vi "Begin.vi"(8 "error in":errorcluster) -> (0 "error out":errorcluster)   [LabVIEW 2016]
doc: "Called before other user functions, this VI is expected to open initial I/O refnums, load in file data, and do all program initialization. Notice that the <B>error out</B> terminal is simply used for data flow. Wiring it to other structures or subVIs ensures that this VI runs first."
uses:
  <vilib>/Rock Robotics/SystemInterfaces/DIO/FPGA_DIOPWMChannel.ctl
  <vilib>/Rock Robotics/WPI/SafetyOutput/WPI_SafetyOutputConfigMenu.ctl
  <vilib>/Rock Robotics/WPI/DriverStation/WPI_DriverStationRobotMode2.ctl
  <vilib>/Rock Robotics/WPI/Joystick/WPI_JoystickDeviceEnum.ctl
  <vilib>/Rock Robotics/SystemInterfaces/DIO/FPGA_DIOChannel.ctl
  <vilib>/Rock Robotics/WPI/Encoder/WPI_EncoderType.ctl
  NI WPI/WPI_SerialPort_USB.ctl
  <vilib>/Rock Robotics/WPI/ThirdParty/CanMotor/TalonSRX/WPI_CANTalonSRX_APIControlMode.ctl
  <vilib>/Rock Robotics/WPI/Solenoid/WPI_SolenoidChannel.ctl
  <vilib>/Rock Robotics/SystemInterfaces/i2clib/i2c_bus.ctl
  <vilib>/Rock Robotics/WPI/Solenoid/WPI_SolenoidValue.ctl
  Robot Global Data.vi
  <vilib>/Rock Robotics/Network Tables/NT Write String Array.vi
  <vilib>/Rock Robotics/WPI/Counter/WPI_CounterDigitalInputToDigitalSource.vi
  navX Library v2/IO/Open/Z900_navX_Open_Serial.vi
  <vilib>/Rock Robotics/WPI/Solenoid/WPI_SolenoidOpenSingle.vi
  <vilib>/Rock Robotics/WPI/MotorControl/WPI_MotorControlOpen VictorSP.vi
  <vilib>/Rock Robotics/WPI/RobotDrive/WPI_RobotDriveOpen4MotorWithVictorSP.vi
  <vilib>/Rock Robotics/WPI/Solenoid/WPI_SolenoidSetEnum.vi
  navX Library v2/navX Library v2.lvlib
  NI WPI/NI WPI Serial USB.lvlib
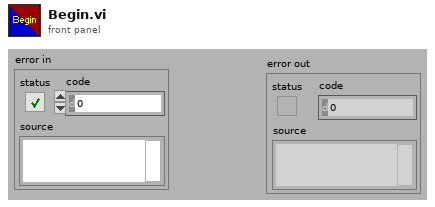
[diagram p1: front panel]
types:
  T1 = typedef "FPGA_DIOChannel.ctl" = enum8{"DIO 0", "DIO 1", "DIO 2", "DIO 3", "DIO 4", "DIO 5", "DIO 6", "DIO 7", "DIO 8", "DIO 9", "DIO MXP 0", "DIO MXP 1", "DIO MXP 2", "DIO MXP 3", "DIO MXP 4", "DIO MXP 5", "DIO MXP 6", "DIO MXP 7", "DIO MXP 8", "DIO MXP 9", "DIO MXP 10", "DIO MXP 11", "DIO MXP 12", "DIO MXP 13", "DIO MXP 14", "DIO MXP 15", "SPI Port CS1", "SPI Port CS2", "SPI Port CS3", "SPI Port MISO", "SPI Port MOSI", "Invalid"}
  T2 = typedef "WPI_SolenoidValue.ctl" = enum16{"Off", "On", "Forward", "Reverse"}
  T3 = typedef "i2c_bus.ctl" = enum16{"I2C On-Board", "I2C MXP", "Invalid"}
  T4 = typedef "WPI_SolenoidChannel.ctl" = enum8{"Solenoid 0", "Solenoid 1", "Solenoid 2", "Solenoid 3", "Solenoid 4", "Solenoid 5", "Solenoid 6", "Solenoid 7", "Invalid"}
  T5 = typedef "FPGA_DIOPWMChannel.ctl" = enum8{"PWM 0", "PWM 1", "PWM 2", "PWM 3", "PWM 4", "PWM 5", "PWM 6", "PWM 7", "PWM 8", "PWM 9", "PWM MXP 0", "PWM MXP 1", "PWM MXP 2", "PWM MXP 3", "PWM MXP 4", "PWM MXP 5", "PWM MXP 6", "PWM MXP 7", "PWM MXP 8", "PWM MXP 9", "Invalid"}
  T6 = typedef "WPI_JoystickDeviceEnum.ctl" = enum16{"USB 0", "USB 1", "USB 2", "USB 3", "USB 4", "USB 5"}
  T7 = typedef "WPI_CANTalonSRX_APIControlMode.ctl" = enum8{"Percent VBus", "Speed", "Position", "Slave", "Unchanged / Invalid", "Voltage Compensation", "Current", "Motion Profile", "Motion Magic"}
  T8 = typedef "NI WPI Serial USB.lvlib/WPI_SerialPort_USB.ctl" = enum16{"Onboard RS-232", "MXP TTL", "USB"}
  T9 = typedef "WPI_EncoderType.ctl" = enum16{"1x", "2x", "4x"}
  T10 = typedef "WPI_DriverStationRobotMode2.ctl" = enum16{"Autonomous Disabled", "Autonomous Enabled", "Teleop Disabled", "Teleop Enabled", "Disconnected", "Finish", "Test Disabled", "Test Enabled", "Emergency Stopped"}
  T11 = typedef "WPI_SafetyOutputConfigMenu.ctl" = enum16{"Enable", "Disable"}
  T12 = typedef "WPI_JoystickDevRef.ctl" = cluster{"Device":T6}
  T13 = typedef "WPI_I2CDevRef.ctl" = cluster{"DevStatus":errorcluster, "Device Address":u8, "Handle":i32, "I2C Bus":T3}
  T14 = typedef "WPI_MotorControlDeviceRef.ctl" = cluster{"DeviceStatus":errorcluster, "Type":T15, "PWM":cluster{"PWM Channel":T5, "DeadBand":T16}, "CAN":cluster{"Device Number":u8, "SetOutput VI Ref":variant, "GetOutput VI Ref":variant, "Enable VI Ref":variant, "Disable VI Ref":variant, "Data":variant}, "Invert":bool}
  T15 = typedef "WPI_MotorControlType.ctl" = enum16{"PWM", "CAN"}
  T16 = typedef "WPI_PWMDeadband.ctl" = cluster{"Name":string, "maxPositivePwm":i32, "minPositivePwm":i32, "centerPwm":i32, "maxNegativePwm":i32, "minNegativePwm":i32, "angularRange":u16}
  T17 = typedef "WPI_RobotDriveDevRef.ctl" = cluster{"DevStatus":errorcluster, "Motors[]":T14[], "Square Inputs":bool, "Max Output":dbl}
  T18 = typedef "WPI_DigitalInputDevRef.ctl" = cluster{"DevStatus":errorcluster, "DIO Channel":T1}
  T19 = typedef "FPGA_CounterEncoderSourceConvertionLVSourceType.ctl" = cluster{"DevStatus":errorcluster, "AnalogTriggerMode?":bool, "DigitalMode":cluster{"DIO Channel":T20}, "AnalogTriggerMode":cluster{"AnalogTriggerIndex":T21, "OutputType":T22}}
  T20 = typedef "FPGA_DIODigitalSourceChannel.ctl" = enum8{"DIO 0", "DIO 1", "DIO 2", "DIO 3", "DIO 4", "DIO 5", "DIO 6", "DIO 7", "DIO 8", "DIO 9", "DIO MXP 0", "DIO MXP 1", "DIO MXP 2", "DIO MXP 3", "DIO MXP 4", "DIO MXP 5", "DIO MXP 6", "DIO MXP 7", "DIO MXP 8", "DIO MXP 9", "DIO MXP 10", "DIO MXP 11", "DIO MXP 12", "DIO MXP 13", "DIO MXP 14", "DIO MXP 15", "Disabled"}
  T21 = typedef "FPGA_AnalogTriggerIndex.ctl" = enum8{"Trig 0", "Trig 1", "Trig 2", "Trig 3", "Trig 4", "Trig 5", "Trig 6", "Trig 7", "Invalid"}
  T22 = typedef "FPGA_AnalogTriggerOutType.ctl" = enum16{"InWindow", "TriggerState", "Rising", "Falling"}
  T23 = typedef "WPI_EncoderDevRef.ctl" = cluster{"DevStatus":errorcluster, "EncoderIndex":T24, "CounterIndex":T25, "DistancePerCount":dbl, "Decoding Type":T9}
  T24 = typedef "FPGA_EncoderIdx.ctl" = enum8{"Enc 0", "Enc 1", "Enc 2", "Enc 3", "Enc 4", "Enc 5", "Enc 6", "Enc 7", "Invalid"}
  T25 = typedef "FPGA_CounterCtrSystemIndex.ctl" = enum8{"Ctr 0", "Ctr 1", "Ctr 2", "Ctr 3", "Ctr 4", "Ctr 5", "Ctr 6", "Ctr 7", "Invalid"}
  T26 = typedef "navX Library v2.lvlib/Z900_navX_DeviceTypeDef.ctl" = cluster{"Interface":cluster{"Protocol":T27, "Update Rate (4Hz-100Hz)":u8, "navX Open TypeDef":variant}, "Notify Packet":refnum<notifier>, "Loop VI Refnum":refnum<vi>, "Ready to Close Occurrence Refnum":refnum<k4>}
  T27 = typedef "navX Library v2.lvlib/Z900_navX_ProtocolTypeDef.ctl" = enum16{"SERIAL", "I2C", "SPI"}
  T28 = typedef "WPI_SolenoidDevRef.ctl" = cluster{"DevStatus":errorcluster, "Pneumatics Control Module":u8, "Forward Solenoid Channel":T4, "Reverse Solenoid Channel":T4}
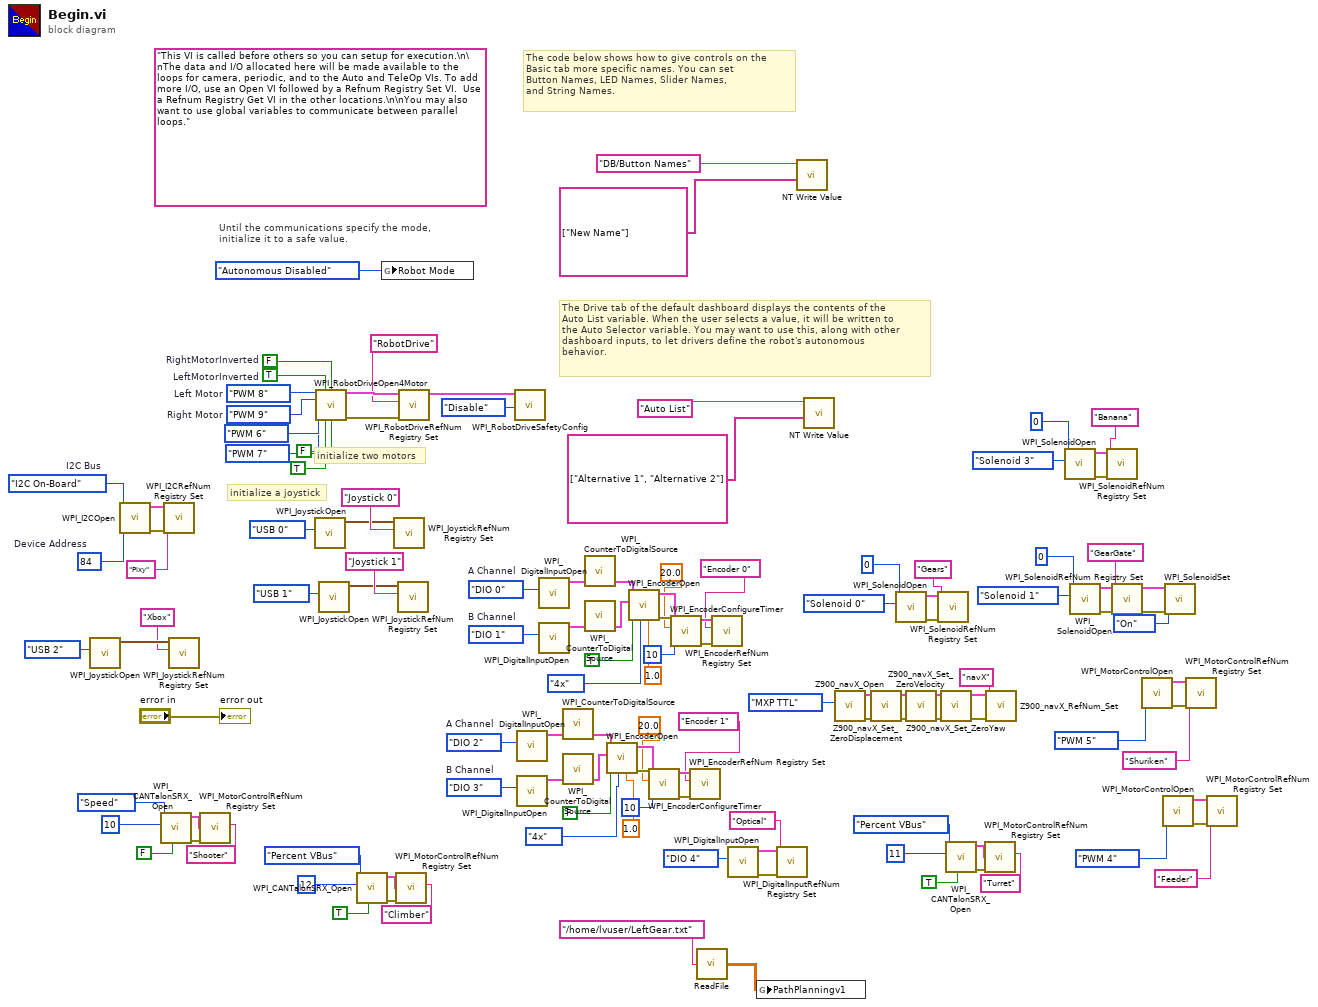
[diagram p0: block diagram]
diagram:
  w14 = u8 84  # Device Address
  w15 = i2c_bus."I2C On-Board"  # I2C Bus
  w88 = FPGA_DIOChannel."DIO 3"  # B Channel
  w87 = FPGA_DIOChannel."DIO 2"  # A Channel
  w104 = FPGA_DIOChannel."DIO 1"  # B Channel
  w103 = FPGA_DIOChannel."DIO 0"  # A Channel
  (unwired) "This VI is called before others so you can setup for execution.\n\nThe data and I/O allocated here will be made available to the loops for camera, periodic, and to the Auto and TeleOp VIs. To add more I/O, use an Open VI followed by a Refnum Registry Set VI.  Use a Refnum Registry Get VI in the other locations.\n\nYou may also want to use global variables to communicate between parallel loops."
  w119 = FPGA_DIOPWMChannel."PWM 9"  # Right Motor
  w120 = FPGA_DIOPWMChannel."PWM 8"  # Left Motor
  w124 = TRUE  # LeftMotorInverted
  w125 = FALSE  # RightMotorInverted
  # "The Drive tab of the default dashboard displays the contents of the\nAuto List variable. When the user selects a value, it will be written to\nthe Auto Selector variable. You may want to use this, along with other\ndashboard inputs, to let drivers define the robot's autonomous\nbehavior."
  # "The code below shows how to give controls on the\nBasic tab more specific names. You can set\nButton Names, LED Names, Slider Names,\nand String Names."
  # "initialize a joystick"
  # "Until the communications specify the mode,\ninitialize it to a safe value."
  # "initialize two motors"
  n1 = call <vilib>:"WPI_JoystickOpen.vi"("JoystickDevice"=WPI_JoystickDeviceEnum."USB 2") -> ("JoystickDevRef"=w28:T12)  [unwired: 10 in]
  n2 = call <vilib>:"WPI_I2COpen.vi"("Device Address"=w14, "I2C Bus"=w15) -> ("error out"=w13:errorcluster, "I2CDevRef"=w12:T13)  [unwired: 8 in]
  n3 = call <vilib>:"WPI_CANTalonSRX_Open.vi"("Invert"=FALSE, "Device Number"=10, "Control Mode"=WPI_CANTalonSRX_APIControlMode."Speed") -> ("error out"=w55:errorcluster, "CAN Talon SRX Ref"=w56:T14)  [unwired: 7 in]
  n4 = call <vilib>:"WPI_I2CRefNum Registry Set.vi"("error in (no error)"=w13, "refnum name"="Pixy", "I2CDevRef"=w12) -> ()  [unwired: 7 in, 2 out]
  n5 = call <vilib>:"WPI_JoystickRefNum Registry Set.vi"("refnum name"="Xbox", "JoystickDevRef"=w28) -> ()  [unwired: 8 in, 2 out]
  n6 = call <vilib>:"WPI_MotorControlRefNum Registry Set.vi"("error in (no error)"=w55, "refnum name"="Shooter", "MotorControlDevRef"=w56) -> ()  [unwired: 7 in, 2 out]
  n7 = call <vilib>:"WPI_JoystickOpen.vi"("JoystickDevice"=WPI_JoystickDeviceEnum."USB 0") -> ("JoystickDevRef"=w114:T12)  [unwired: 10 in]
  n8 = call-poly <vilib>:"WPI_RobotDriveOpen4Motor.vi"("Rear Left Motor"=w120, "Rear Left Motor Inverted"=w124, "Rear Right Motor Inverted"=w125, "Rear Right Motor"=w119, "Front Left Motor"=FPGA_DIOPWMChannel."PWM 6", "Front Right Motor"=FPGA_DIOPWMChannel."PWM 7", "Front Left Motor Inverted"=TRUE, "Front Right Motor Inverted"=FALSE) -> ("RobotDriveDevRef"=w123:T17, "error out"=w121:errorcluster)  [unwired: 6 in]
  n9 = call <vilib>:"WPI_JoystickOpen.vi"("JoystickDevice"=WPI_JoystickDeviceEnum."USB 1") -> ("JoystickDevRef"=w106:T12)  [unwired: 10 in]
  n10 = call <vilib>:"WPI_CANTalonSRX_Open.vi"("Invert"=TRUE, "Device Number"=12, "Control Mode"=WPI_CANTalonSRX_APIControlMode."Percent VBus") -> ("error out"=w49:errorcluster, "CAN Talon SRX Ref"=w50:T14)  [unwired: 7 in]
  n11 = global write "Robot Global Data.vi" "Robot Mode"(WPI_DriverStationRobotMode2."Autonomous Disabled" ("Robot Mode")) -> ()
  n12 = call <vilib>:"WPI_JoystickRefNum Registry Set.vi"("refnum name"="Joystick 0", "JoystickDevRef"=w114) -> ()  [unwired: 8 in, 2 out]
  n13 = call <vilib>:"WPI_MotorControlRefNum Registry Set.vi"("error in (no error)"=w49, "refnum name"="Climber", "MotorControlDevRef"=w50) -> ()  [unwired: 7 in, 2 out]
  n14 = call <vilib>:"WPI_JoystickRefNum Registry Set.vi"("refnum name"="Joystick 1", "JoystickDevRef"=w106) -> ()  [unwired: 8 in, 2 out]
  n15 = call <vilib>:"WPI_RobotDriveRefNum Registry Set.vi"("error in (no error)"=w121, "refnum name"="RobotDrive", "RobotDriveDevRef"=w123) -> ("RobotDriveDevRef"=w118:T17)  [unwired: 1 in, 7 out]
  n16 = call <vilib>:"WPI_RobotDriveSafetyConfig.vi"("mode"=WPI_SafetyOutputConfigMenu."Disable", "RobotDriveDevRef"=w118) -> ()  [unwired: 8 in, 2 out]
  n17 = call <vilib>:"WPI_DigitalInputOpen.vi"("DIO Channel"=w87) -> ("DigitalInputDevRef"=w84:T18)  [unwired: 1 in, 9 out]
  n18 = call <vilib>:"WPI_DigitalInputOpen.vi"("DIO Channel"=w88) -> ("DigitalInputDevRef"=w85:T18)  [unwired: 1 in, 9 out]
  n19 = call <vilib>:"WPI_DigitalInputOpen.vi"("DIO Channel"=w103) -> ("DigitalInputDevRef"=w100:T18)  [unwired: 1 in, 9 out]
  n20 = call <vilib>:"WPI_DigitalInputOpen.vi"("DIO Channel"=w104) -> ("DigitalInputDevRef"=w101:T18)  [unwired: 1 in, 9 out]
  n21 = call-poly <vilib>:"WPI_CounterToDigitalSource.vi"("DigitalInputDevRef"=w84) -> ("Digital Source"=w83:T19)  [unwired: 6 out]
  n22 = call-poly <vilib>:"WPI_CounterToDigitalSource.vi"("DigitalInputDevRef"=w85) -> ("Digital Source"=w86:T19)  [unwired: 6 out]
  n23 = call-poly <vilib>:"WPI_CounterToDigitalSource.vi"("DigitalInputDevRef"=w100) -> ("Digital Source"=w99:T19)  [unwired: 6 out]
  n24 = call-poly <vilib>:"WPI_CounterToDigitalSource.vi"("DigitalInputDevRef"=w101) -> ("Digital Source"=w102:T19)  [unwired: 6 out]
  n25 = call <vilib>:"WPI_EncoderOpen.vi"("DistancePerCount"=1.0, "Decoding Type"=WPI_EncoderType."4x", "Invert Direction (False)"=FALSE, "BSource"=w86, "ASource"=w83) -> ("error out"=w81:errorcluster, "EncoderDevRef"=w80:T23)  [unwired: 3 in, 2 out]
  n26 = call <vilib>:"WPI_EncoderOpen.vi"("DistancePerCount"=1.0, "Decoding Type"=WPI_EncoderType."4x", "Invert Direction (False)"=TRUE, "BSource"=w102, "ASource"=w99) -> ("error out"=w95:errorcluster, "EncoderDevRef"=w94:T23)  [unwired: 3 in, 2 out]
  n27 = call <vilib>:"WPI_EncoderConfigureTimer.vi"("error in (no error)"=w81, "Number Samples to Average"=u8 10, "Minimum Rate"=20.0, "EncoderDevRef"=w80) -> ("error out"=w77:errorcluster, "EncoderDevRef"=w76:T23)  [unwired: 6 in]
  n28 = call <vilib>:"WPI_EncoderConfigureTimer.vi"("error in (no error)"=w95, "Number Samples to Average"=u8 10, "Minimum Rate"=20.0, "EncoderDevRef"=w94) -> ("error out"=w91:errorcluster, "EncoderDevRef"=w90:T23)  [unwired: 6 in]
  n29 = call <vilib>:"WPI_EncoderRefNum Registry Set.vi"("error in (no error)"=w77, "refnum name"="Encoder 1", "EncoderDevRef"=w76) -> ()  [unwired: 7 in, 2 out]
  n30 = call "ReadFile.vi"("Name"="/home/lvuser/LeftGear.txt") -> ("Array - Numeric"=w8:dbl[][])
  n31 = call <vilib>:"WPI_EncoderRefNum Registry Set.vi"("error in (no error)"=w91, "refnum name"="Encoder 0", "EncoderDevRef"=w90) -> ()  [unwired: 7 in, 2 out]
  n32 = call <vilib>:"WPI_DigitalInputOpen.vi"("DIO Channel"=FPGA_DIOChannel."DIO 4") -> ("error out"=w4:errorcluster, "DigitalInputDevRef"=w3:T18)  [unwired: 9 in]
  n33 = global write "Robot Global Data.vi" "PathPlanningv1"(w8) -> ()
  n34 = call <vilib>:"WPI_DigitalInputRefNum Registry Set.vi"("error in (no error)"=w4, "refnum name"="Optical", "DigitalInputDevRef"=w3) -> ()  [unwired: 7 in, 2 out]
  n35 = call-poly <vilib>:"NT Write Value.vi"("String Array"=string[] ["New Name"], "Name"="DB/Button Names") -> ()  [unwired: 9 in, 1 out]
  n36 = call-poly <vilib>:"NT Write Value.vi"("String Array"=string[] ["Alternative 1", "Alternative 2"], "Name"="Auto List") -> ()  [unwired: 9 in, 1 out]
  n37 = call-poly "Z900_navX_Open.vi"("Serial Port"=WPI_SerialPort_USB."MXP TTL") -> ("error out"=w63:errorcluster, "navX Device"=w68:T26)  [unwired: 9 in]
  n38 = call "Z900_navX_Set_ZeroDisplacement.vi"("error in (no error)"=w63, "navX Device"=w68) -> ("error out"=w62:errorcluster, "navX Device"=w67:T26)  [unwired: 8 in]
  n39 = call-poly <vilib>:"WPI_SolenoidOpen.vi"("Solenoid Channel"=WPI_SolenoidChannel."Solenoid 0", "Pneumatics Control Module (0)"=u8 0) -> ("error out"=w48:errorcluster, "SolenoidDevRef"=w47:T28)  [unwired: 8 in]
  n40 = call "Z900_navX_Set_ZeroVelocity.vi"("error in (no error)"=w62, "navX Device"=w67) -> ("error out"=w61:errorcluster, "navX Device"=w66:T26)  [unwired: 8 in]
  n41 = call <vilib>:"WPI_SolenoidRefNum Registry Set.vi"("error in (no error)"=w48, "refnum name"="Gears", "SolenoidDevRef"=w47) -> ()  [unwired: 7 in, 2 out]
  n42 = call "Z900_navX_Set_ZeroYaw.vi"("error in (no error)"=w61, "navX Device"=w66) -> ("error out"=w64:errorcluster, "navX Device"=w65:T26)  [unwired: 8 in]
  n43 = call <vilib>:"WPI_CANTalonSRX_Open.vi"("Invert"=TRUE, "Device Number"=11, "Control Mode"=WPI_CANTalonSRX_APIControlMode."Percent VBus") -> ("error out"=w38:errorcluster, "CAN Talon SRX Ref"=w39:T14)  [unwired: 7 in]
  n44 = call <vilib>:"WPI_MotorControlRefNum Registry Set.vi"("error in (no error)"=w38, "refnum name"="Turret", "MotorControlDevRef"=w39) -> ()  [unwired: 7 in, 2 out]
  n45 = call "Z900_navX_RefNum_Set.vi"("error in (no error)"=w64, "refnum name"="navX", "navX Device"=w65) -> ()  [unwired: 7 in, 2 out]
  n46 = call-poly <vilib>:"WPI_SolenoidOpen.vi"("Solenoid Channel"=WPI_SolenoidChannel."Solenoid 3", "Pneumatics Control Module (0)"=u8 0) -> ("error out"=w20:errorcluster, "SolenoidDevRef"=w19:T28)  [unwired: 8 in]
  n47 = call-poly <vilib>:"WPI_SolenoidOpen.vi"("Solenoid Channel"=WPI_SolenoidChannel."Solenoid 1", "Pneumatics Control Module (0)"=u8 0) -> ("error out"=w33:errorcluster, "SolenoidDevRef"=w32:T28)  [unwired: 8 in]
  n48 = call <vilib>:"WPI_SolenoidRefNum Registry Set.vi"("error in (no error)"=w20, "refnum name"="Banana", "SolenoidDevRef"=w19) -> ()  [unwired: 7 in, 2 out]
  n49 = call <vilib>:"WPI_SolenoidRefNum Registry Set.vi"("error in (no error)"=w33, "refnum name"="GearGate", "SolenoidDevRef"=w32) -> ("error out"=w7:errorcluster, "SolenoidDevRef"=w6:T28)  [unwired: 7 in]
  n50 = call-poly <vilib>:"WPI_MotorControlOpen.vi"("PWM Channel"=FPGA_DIOPWMChannel."PWM 5") -> ("error out"=w37:errorcluster, "MotorControlDeviceRef"=w36:T14)  [unwired: 9 in]
  n51 = call-poly <vilib>:"WPI_MotorControlOpen.vi"("PWM Channel"=FPGA_DIOPWMChannel."PWM 4") -> ("error out"=w25:errorcluster, "MotorControlDeviceRef"=w24:T14)  [unwired: 9 in]
  n52 = call-poly <vilib>:"WPI_SolenoidSet.vi"("error in (no error)"=w7, "Value"=WPI_SolenoidValue."On", "SolenoidDevRef"=w6) -> ()  [unwired: 7 in, 2 out]
  n53 = call <vilib>:"WPI_MotorControlRefNum Registry Set.vi"("error in (no error)"=w37, "refnum name"="Shuriken", "MotorControlDevRef"=w36) -> ()  [unwired: 7 in, 2 out]
  n54 = call <vilib>:"WPI_MotorControlRefNum Registry Set.vi"("error in (no error)"=w25, "refnum name"="Feeder", "MotorControlDevRef"=w24) -> ()  [unwired: 7 in, 2 out]
  "error out" <- "error in"
